vi "Names and Default Values.vi"() -> (3 "Names and Default Values":T2={"Signal"={"Sample Rate"={"name"="SignalSampleRate", "default"=51200.0}, "Signal Type"={"name"="SignalType", "signal type"=enum."None"}, "Amplitude"={"name"="SignalAmplitude", "default"=1.0}, "Offset"={"name"="SignalOffset", "default"=0.0}}, "Function"={"Info"={"name"="FunctionInfo", "default"=variant}, "Type"={"name"="Type", "default"=0}, "Frequency"={"name"="Frequency", "default"=1000.0}, "Phase"={"name"="Phase", "default"=0.0}}, "Continuous Sweep"={"Info"={"name"="ContinuousSweepInfo", "default"=variant}, "Start"={"name"="Start", "default"=100.0}, "Stop"={"name"="Stop", "default"=10000.0}, "Duration"={"name"="Duration", "default"=1.0}, "Profile"={"name"="Profile", "default"=enum."Logarithmic"}}, "Discrete Sweep"={"Info"={"name"="DiscreteSweepInfo", "default"=variant}, "Start"={"name"="Start", "default"=100.0}, "Stop"={"name"="Stop", "default"=10000.0}, "Cycles"={"name"="Cycles", "default"=10.0}, "Time"={"name"="Time", "default"=0.01}, "Spacing"={"name"="Spacing", "default"=enum."Logarithmic"}, "Steps"={"name"="Steps", "default"=100}}, "Multitone"={"Info"={"name"="MultitoneInfo", "multitone info"=[{"frequency"=1000.0, "amplitude"=1.0, "phase"=0.0}, {"frequency"=2000.0, "amplitude"=1.0, "phase"=50.0}, {"frequency"=3000.0, "amplitude"=1.0, "phase"=150.0}, {"frequency"=4000.0, "amplitude"=1.0, "phase"=250.0}]}}, "Noise"={"Info"={"name"="NoiseInfo", "default"=variant}, "Type"={"name"="Type", "default"=0}, "Amplitude PDF"={"name"="PDF", "default"=enum."Gaussian"}, "Level"={"name"="Level", "default"=-1.0}, "Seed"={"name"="Seed", "default"=-1}}, "Configuration"={"Min Frequency"={"name"="SignalSampleRate", "default"=20.0}, "Max Frequency"={"name"="Maximum Frequency", "default"=20000.0}, "Max Amplitude"={"name"="SignalAmplitude", "default"=2.0}}} {"Noise"."Type"."default" items=["White noise", "Pink noise", "Periodic random noise"]; "Multitone"."Info"."multitone info"."phase" format="%#.1f°"; "Multitone"."Info"."multitone info"."amplitude" format="%#_4g"; "Multitone"."Info"."multitone info"."frequency" format="%#_5p Hz"; "Discrete Sweep"."Steps"."default" min=1; "Function"."Type"."default" items=["Sine", "Triangle", "Square", "Sawtooth"]})   [LabVIEW 2017, in "Test Signal Configuration.xctl"]
uses:
  <vilib>/addons/_XControls/Function Generator Configuration/Test Signal Configuration.xctl
  <vilib>/addons/_XControls/Function Generator Configuration/Controls/signal type.ctl
panel:
  # "fi"
  # "ai"
  # "fi"
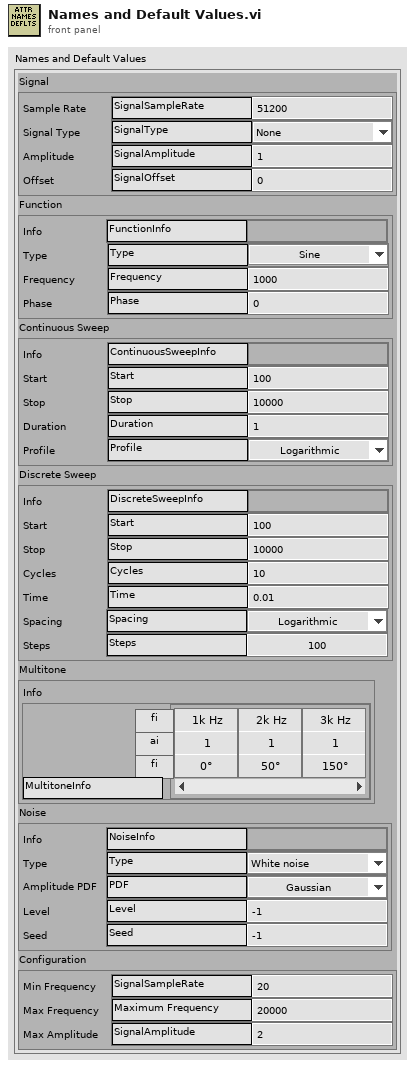
[diagram p1: front panel]
types:
  T1 = typedef "Test Signal Configuration.xctl/signal type.ctl" = enum32{"None", "Tone", "Multitone", "Discrete Sweep", "Continuous Sweep", "Noise"}
  T2 = cluster{"Signal":cluster{"Sample Rate":cluster{"name":string, "default":dbl}, "Signal Type":cluster{"name":string, "signal type":T1}, "Amplitude":cluster{"name":string, "default":dbl}, "Offset":cluster{"name":string, "default":dbl}}, "Function":cluster{"Info":cluster{"name":string, "default":variant}, "Type":cluster{"name":string, "default":u16}, "Frequency":cluster{"name":string, "default":dbl}, "Phase":cluster{"name":string, "default":dbl}}, "Continuous Sweep":cluster{"Info":cluster{"name":string, "default":variant}, "Start":cluster{"name":string, "default":dbl}, "Stop":cluster{"name":string, "default":dbl}, "Duration":cluster{"name":string, "default":dbl}, "Profile":cluster{"name":string, "default":enum16{"Linear", "Logarithmic"}}}, "Discrete Sweep":cluster{"Info":cluster{"name":string, "default":variant}, "Start":cluster{"name":string, "default":dbl}, "Stop":cluster{"name":string, "default":dbl}, "Cycles":cluster{"name":string, "default":dbl}, "Time":cluster{"name":string, "default":dbl}, "Spacing":cluster{"name":string, "default":enum16{"Linear", "Logarithmic"}}, "Steps":cluster{"name":string, "default":i32}}, "Multitone":cluster{"Info":cluster{"name":string, "multitone info":cluster{"frequency":dbl, "amplitude":dbl, "phase":dbl}[]}}, "Noise":cluster{"Info":cluster{"name":string, "default":variant}, "Type":cluster{"name":string, "default":u16}, "Amplitude PDF":cluster{"name":string, "default":enum16{"Gaussian", "Rectangular", "Triangular"}}, "Level":cluster{"name":string, "default":dbl}, "Seed":cluster{"name":string, "default":i32}}, "Configuration":cluster{"Min Frequency":cluster{"name":string, "default":dbl}, "Max Frequency":cluster{"name":string, "default":dbl}, "Max Amplitude":cluster{"name":string, "default":dbl}}}
  T3 = cluster{cluster{"Sample Rate":cluster{"name":string, "default":dbl}, "Signal Type":cluster{"name":string, "signal type":T1}, "Amplitude":cluster{"name":string, "default":dbl}, "Offset":cluster{"name":string, "default":dbl}}, "Function":cluster{"Info":cluster{"name":string, "default":variant}, "Type":cluster{"name":string, "default":u16}, "Frequency":cluster{"name":string, "default":dbl}, "Phase":cluster{"name":string, "default":dbl}}, "Continuous Sweep":cluster{"Info":cluster{"name":string, "default":variant}, "Start":cluster{"name":string, "default":dbl}, "Stop":cluster{"name":string, "default":dbl}, "Duration":cluster{"name":string, "default":dbl}, "Profile":cluster{"name":string, "default":enum16{"Linear", "Logarithmic"}}}, "Discrete Sweep":cluster{"Info":cluster{"name":string, "default":variant}, "Start":cluster{"name":string, "default":dbl}, "Stop":cluster{"name":string, "default":dbl}, "Cycles":cluster{"name":string, "default":dbl}, "Time":cluster{"name":string, "default":dbl}, "Spacing":cluster{"name":string, "default":enum16{"Linear", "Logarithmic"}}, "Steps":cluster{"name":string, "default":i32}}, "Multitone":cluster{"Info":cluster{"name":string, "multitone info":cluster{"frequency":dbl, "amplitude":dbl, "phase":dbl}[]}}, "Noise":cluster{"Info":cluster{"name":string, "default":variant}, "Type":cluster{"name":string, "default":u16}, "Amplitude PDF":cluster{"name":string, "default":enum16{"Gaussian", "Rectangular", "Triangular"}}, "Level":cluster{"name":string, "default":dbl}, "Seed":cluster{"name":string, "default":i32}}, "Configuration":cluster{"Min Frequency":cluster{"name":string, "default":dbl}, "Max Frequency":cluster{"name":string, "default":dbl}, "Max Amplitude":cluster{"name":string, "default":dbl}}}
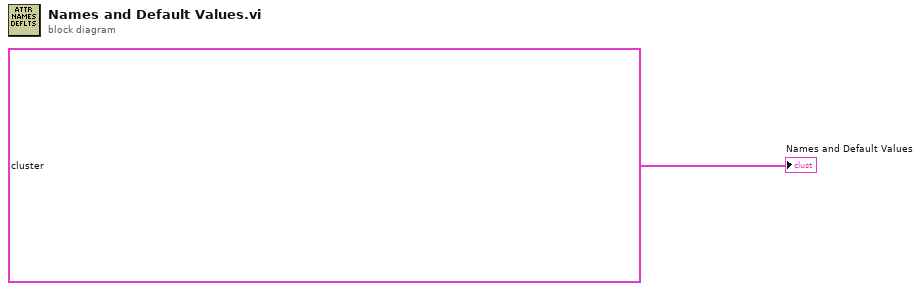
[diagram p0: block diagram]
diagram:
  "Names and Default Values" <- T3 {{"Sample Rate"={"name"="SignalSampleRate", "default"=51200.0}, "Signal Type"={"name"="SignalType", "signal type"=enum."Tone"}, "Amplitude"={"name"="SignalAmplitude", "default"=1.0}, "Offset"={"name"="SignalOffset", "default"=0.0}}, "Function"={"Info"={"name"="FunctionInfo", "default"=variant}, "Type"={"name"="Type", "default"=0}, "Frequency"={"name"="Frequency", "default"=1000.0}, "Phase"={"name"="Phase", "default"=0.0}}, "Continuous Sweep"={"Info"={"name"="ContinuousSweepInfo", "default"=variant}, "Start"={"name"="Start", "default"=100.0}, "Stop"={"name"="Stop", "default"=10000.0}, "Duration"={"name"="Duration", "default"=1.0}, "Profile"={"name"="Profile", "default"=enum."Logarithmic"}}, "Discrete Sweep"={"Info"={"name"="DiscreteSweepInfo", "default"=variant}, "Start"={"name"="Start", "default"=100.0}, "Stop"={"name"="Stop", "default"=10000.0}, "Cycles"={"name"="Cycles", "default"=10.0}, "Time"={"name"="Time", "default"=0.01}, "Spacing"={"name"="Spacing", "default"=enum."Logarithmic"}, "Steps"={"name"="Steps", "default"=100}}, "Multitone"={"Info"={"name"="MultitoneInfo", "multitone info"=[{"frequency"=1000.0, "amplitude"=1.0, "phase"=0.0}, {"frequency"=2000.0, "amplitude"=1.0, "phase"=50.0}, {"frequency"=3000.0, "amplitude"=1.0, "phase"=150.0}, {"frequency"=4000.0, "amplitude"=1.0, "phase"=250.0}]}}, "Noise"={"Info"={"name"="NoiseInfo", "default"=variant}, "Type"={"name"="Type", "default"=0}, "Amplitude PDF"={"name"="PDF", "default"=enum."Gaussian"}, "Level"={"name"="Level", "default"=-1.0}, "Seed"={"name"="Seed", "default"=-1}}, "Configuration"={"Min Frequency"={"name"="Minimum Frequency", "default"=20.0}, "Max Frequency"={"name"="Maximum Frequency", "default"=20000.0}, "Max Amplitude"={"name"="Maximum Amplitude", "default"=2.0}}} ("Names and Default Values")
